vi "DEMO.vi"() -> ()   [LabVIEW 2013]
doc: "Use this template to build a producer/consumer design pattern with events to produce queue items. Use this design pattern instead of the User Interface Event Handler pattern for user interfaces when you want to execute code asynchronously in response to an event without slowing the user interface responsiveness."
uses:
  Command.lvclass/Command.lvclass
  AirCondition.lvclass/AirCondition.lvclass
  RoomLight.lvclass/RoomLight.lvclass
  OutDoorLight.lvclass/OutDoorLight.lvclass
  Television.lvclass/Television.lvclass
  Stereo.lvclass/Stereo.lvclass
  Command.lvclass/ObjectCluster.ctl
  RoomLightCommand.lvclass/RoomLightCommand.lvclass
  OutDoorLightCommand.lvclass/OutDoorLightCommand.lvclass
  AirConditionCommand.lvclass/AirConditionCommand.lvclass
  TelevisionCommand.lvclass/TelevisionCommand.lvclass
  StereoCommand.lvclass/StereoCommand.lvclass
panel:
  out "音響":bool
  out "電視":bool
  out "空調":bool
  out "室外燈":bool
  out "室內燈":bool
  in  "Select":enum16{"室內燈", "室外燈", "空調", "電視", "音響"}(ring) caption="選擇裝置"
  in  "Switch":bool
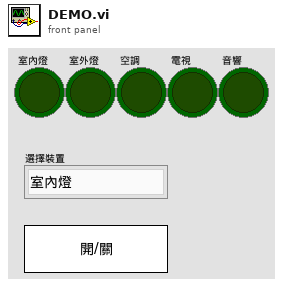
[diagram p1: front panel]
types:
  T1 = typedef "Command.lvclass/ObjectCluster.ctl" = cluster{"AirCondition.lvclass":refnum<class "AirCondition.lvclass">, "RoomLight.lvclass":refnum<class "RoomLight.lvclass">, "OutDoorLight.lvclass":refnum<class "OutDoorLight.lvclass">, "Television.lvclass":refnum<class "Television.lvclass">, "Stereo.lvclass":refnum<class "Stereo.lvclass">}
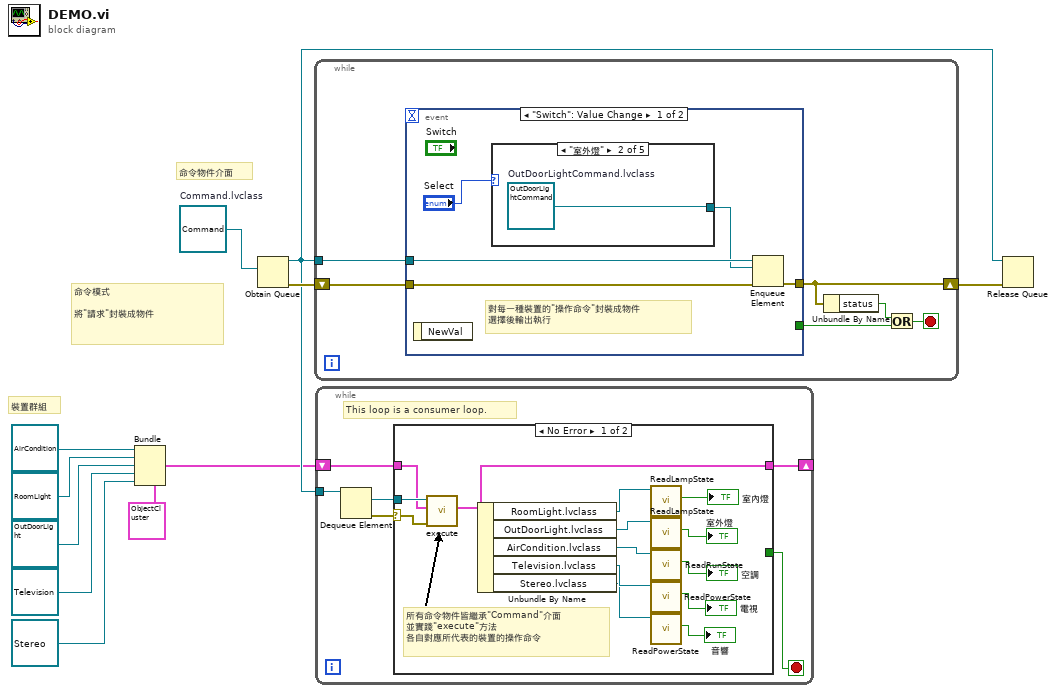
[diagram p0: block diagram]
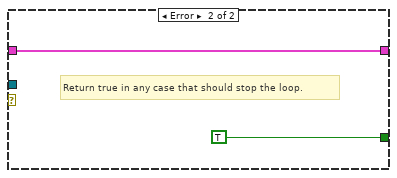
[diagram p2: hidden frame]
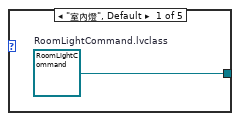
[diagram p3: hidden frame]
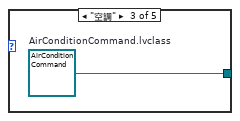
[diagram p4: hidden frame]
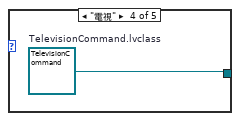
[diagram p5: hidden frame]
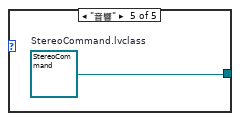
[diagram p6: hidden frame]
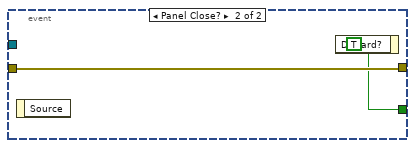
[diagram p7: hidden frame]
diagram:
  w8 = refnum<class "Command.lvclass"> refnum  # Command.lvclass
  # "裝置群組"
  # "命令物件介面"
  # "命令模式\n\n將\"請求\"封裝成物件"
  n1 = Bundle(cluster=T1 {"AirCondition.lvclass"=refnum, "RoomLight.lvclass"=refnum, "OutDoorLight.lvclass"=refnum, "Television.lvclass"=refnum, "Stereo.lvclass"=refnum} ("ObjectCluster"), "AirCondition.lvclass"=refnum<class "AirCondition.lvclass"> refnum, "RoomLight.lvclass"=refnum<class "RoomLight.lvclass"> refnum, "OutDoorLight.lvclass"=refnum<class "OutDoorLight.lvclass"> refnum, "Television.lvclass"=refnum<class "Television.lvclass"> refnum, "Stereo.lvclass"=refnum<class "Stereo.lvclass"> refnum) -> (w2:T1)
  n2 = Obtain Queue(element data type=w8) -> (queue out=w9:refnum<queue>, error out=w11:errorcluster)  [unwired: 4 in, 1 out]
  n3 = while {
    shift-right: [w13] -> w10
    shift-left: w11 -> [w16]
    tunnel: w9 -> [w17]
    stop <- w14 stop-if-true
    n4 = event shown="[0] \"Switch\": Value Change" {
      selector: _ -> [_ _]
      dyn-events: _ -> [_ _]
      timeout: _ -> [_ _]
      tunnel: w17 -> [w22 _]
      tunnel: w16 -> [w21 w29]
      tunnel: [w20 w29] -> w13
      tunnel: [_ w28] -> w15
      event "Switch": Value Change {
        # "對每一種裝置的\"操作命令\"封裝成物件\n選擇後輸出執行"
        n5 = event-data() -> ()  [unwired: 1 in, 1 out]
        n6 = case shown="\"室外燈\"" "Select" {
          tunnel: [w23 w24 w25 w26 w27] -> w18
          frame "室內燈", Default {
            w23 = refnum<class "RoomLightCommand.lvclass"> refnum  # RoomLightCommand.lvclass
          }
          frame "室外燈" {
            w24 = refnum<class "OutDoorLightCommand.lvclass"> refnum  # OutDoorLightCommand.lvclass
          }
          frame "空調" {
            w25 = refnum<class "AirConditionCommand.lvclass"> refnum  # AirConditionCommand.lvclass
          }
          frame "電視" {
            w26 = refnum<class "TelevisionCommand.lvclass"> refnum  # TelevisionCommand.lvclass
          }
          frame "音響" {
            w27 = refnum<class "StereoCommand.lvclass"> refnum  # StereoCommand.lvclass
          }
        }
        n7 = Enqueue Element(queue=w22, element=w18, error in (no error)=w21) -> (error out=w20:errorcluster)  [unwired: 1 in, 2 out]
      }
      event Panel Close? {
        w28 = TRUE ("Discard?")
        n8 = event-data() -> ()  [unwired: 1 in, 1 out]
        n9 = event-data("Discard?"=w28) -> ()  [unwired: 1 in, 1 out]
      }
    }
    n10 = Unbundle By Name(w13) -> ("status"=w12:bool)
    n11 = Or(x=w12, y=w15) -> (x .or. y?=w14:bool)
  }
  n12 = while {
    tunnel: w9 -> [w35]
    shift-right: [w30] -> _
    shift-left: w2 -> [w31]
    stop <- w32 stop-if-true
    # "This loop is a consumer loop."
    n13 = Dequeue Element(queue=w35) -> (element=w33:refnum<class "Command.lvclass">, error out=w34:errorcluster)  [unwired: 2 in, 2 out]
    n14 = case shown="No Error" w34 {
      selector: w34 -> [w47 _]
      tunnel: w33 -> [w49 _]
      tunnel: [_ TRUE] -> w32
      tunnel: w31 -> [w48 w50]
      tunnel: [w46 w50] -> w30
      frame No Error {
        # "所有命令物件皆繼承\"Command\"介面\n並實踐\"execute\"方法\n各自對應所代表的裝置的操作命令"
        n15 = call-dynamic "execute.vi"("error in (no error)"=w47, "ObjectCluster"=w48, "Command in"=w49) -> ("ObjectCluster Out"=w46:T1)  [unwired: 6 in, 2 out]
        n16 = Unbundle By Name(w46) -> ("RoomLight.lvclass"=w45:refnum<class "RoomLight.lvclass">, "OutDoorLight.lvclass"=w44:refnum<class "OutDoorLight.lvclass">, "AirCondition.lvclass"=w43:refnum<class "AirCondition.lvclass">, "Television.lvclass"=w42:refnum<class "Television.lvclass">, "Stereo.lvclass"=w41:refnum<class "Stereo.lvclass">)
        n17 = call-dynamic "ReadLampState.vi"("RoomLight in"=w45) -> ("LampState"=→"室內燈":bool)  [unwired: 8 in, 2 out]
        n18 = call-dynamic "ReadLampState.vi"("OutDoorLight in"=w44) -> ("LampState"=→"室外燈":bool)  [unwired: 8 in, 2 out]
        n19 = call-dynamic "ReadRunState.vi"("AirCondition in"=w43) -> ("RunState"=→"空調":bool)  [unwired: 8 in, 2 out]
        n20 = call-dynamic "ReadPowerState.vi"("Television in"=w42) -> ("PowerState"=→"電視":bool)  [unwired: 8 in, 2 out]
        n21 = call-dynamic "ReadPowerState.vi"("Stereo in"=w41) -> ("PowerState"=→"音響":bool)  [unwired: 8 in, 2 out]
      }
      frame Error {
        # "Return true in any case that should stop the loop."
      }
    }
  }
  n22 = Release Queue(queue=w9, error in (no error)=w10) -> ()  [unwired: 1 in, 3 out]
